vi "Test2.vi"() -> ()   [LabVIEW 2018]
uses:
  <vilib>/Skyline/TestMonitor/Shared/typedefs/Status Type.ctl
  <vilib>/Skyline/TestMonitor/Test Result/Create Test Result (Single).vi
  <vilib>/Skyline/TestMonitor/Test Result/Update Test Result (Single).vi
  <vilib>/Skyline/TestMonitor/Test Result/NI SystemLink Test Result.lvclass
  logger/Logger.lvclass
  <vilib>/Skyline/TestMonitor/Shared/NI SystemLink Test Monitor.lvlib
panel:
  out "current time":timestamp
  out "Program":string
  out "Serial Number":string
  out "error out":errorcluster
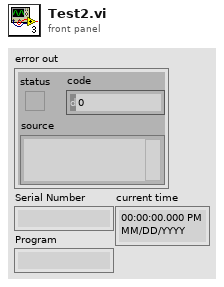
[diagram p1: front panel]
types:
  T1 = typedef "NI SystemLink Test Monitor.lvlib/Status Type.ctl" = enum16{"Failed", "Passed", "Looping", "Skipped", "Custom", "Done", "Running", "Waiting", "Terminated", "Errored", "Timed Out", "None"}
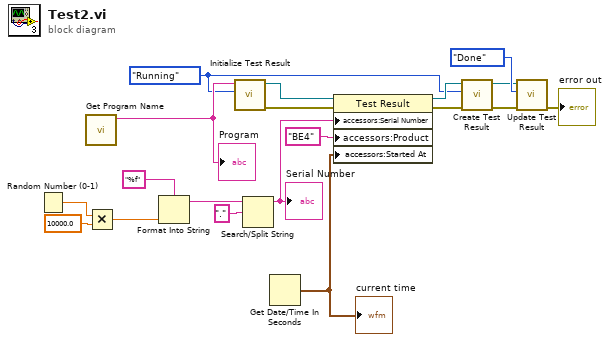
[diagram p0: block diagram]
diagram:
  w2 = Status_Type."Running" ("status type")
  n1 = Random Number (0-1)() -> (number: 0 to 1=w14:dbl)
  n2 = call "Get Program Name.vi"() -> ("String"=w19:string)  [unwired: 11 in]
  "Program" <- w19
  n3 = Multiply(x=w14, y=10000.0) -> (x*y=w12:dbl)
  n4 = Format Into String(format string="%f", w12) -> (resulting string=w16:string)  [unwired: 2 in, 1 out]
  n5 = call <vilib>:"Initialize Test Result.vi"("status type (Running)"=w2, "program name"=w19) -> ("error out"=w9:errorcluster, "test result"=w18:refnum<class "NI SystemLink Test Result.lvclass">)  [unwired: 8 in]
  n6 = Search/Split String(string=w16, search string/char (-)=".") -> (substring before match=w11:string)  [unwired: 1 in, 2 out]
  "Serial Number" <- w11
  n7 = Get Date/Time In Seconds() -> (seconds since 1Jan1904=w1:timestamp)
  "current time" <- w1
  n8 = property class="Test Result"(reference=w18, error in=w9, "accessors:Serial Number"=w11, "accessors:Product"="BE4" ("Product"), "accessors:Started At"=w1) -> (reference out=w10:refnum<class "NI SystemLink Test Result.lvclass">, error out=w8:errorcluster)
  n9 = call-poly <vilib>:"Create Test Result.vi"("error in (no error)"=w8, "status type"=w2, "test result out"=w10) -> ("error out"=w4:errorcluster, "test result out"=w5:refnum<class "NI SystemLink Test Result.lvclass">)  [unwired: 7 in]
  n10 = call-poly <vilib>:"Update Test Result.vi"("error in (no error)"=w4, "status type"=Status_Type."Done", "test result out"=w5) -> ("error out"=→"error out":errorcluster)  [unwired: 7 in, 1 out]
